vi "find_analog_data.vi"(10 "Needle":string, 11 "Haystack":T1[](array[typedef])) -> (0 "Index":i32, 1 "Found?":bool, 2 "Needle Out":T1)   [LabVIEW 2017]
uses:
  Box/Annular Flow/Jason/LabVIEW 2017/Input Channel Lists/analog_data.ctl
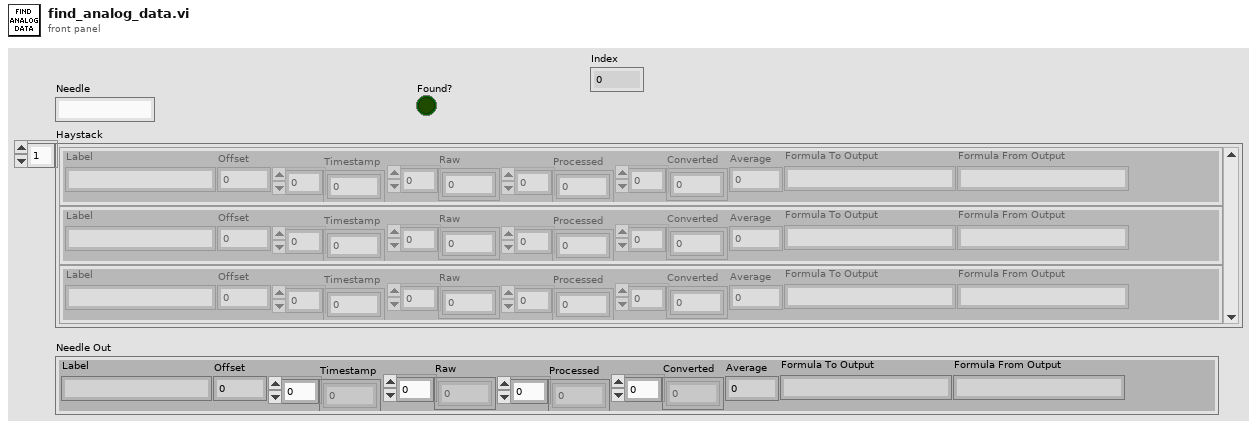
[diagram p1: front panel]
types:
  T1 = typedef "analog_data.ctl" = cluster{"Label":string, "Offset":dbl, "Timestamp":dbl[], "Raw":dbl[], "Processed":dbl[], "Converted":dbl[], "Average":dbl, "Formula To Output":string, "Formula From Output":string}
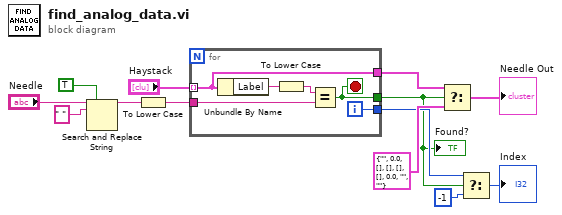
[diagram p0: block diagram]
diagram:
  n1 = Search and Replace String(replace all?=TRUE ("replace all? (F)"), input string="Needle", search string=" ") -> (result string=w9:string)  [unwired: 5 in, 3 out]
  n2 = To Lower Case(string=w9) -> (all lower case string=w8:string)
  n3 = for {
    tunnel: "Haystack" -> [w15] mode=indexing
    tunnel: w8 -> [w17]
    tunnel: [w16] -> w2
    tunnel: [w15] -> w7
    tunnel: [w14] -> w3
    i -> [w14]
    stop <- w16 stop-if-true
    n4 = Unbundle By Name(w15) -> ("Label"=w19:string)
    n5 = To Lower Case(string=w19) -> (all lower case string=w18:string)
    n6 = Equal?(x=w18, y=w17) -> (x = y?=w16:bool)
  }
  "Found?" <- w2
  n7 = Select(t=w7, s=w2, f=T1 {"Label"="", "Offset"=0.0, "Timestamp"=[], "Raw"=[], "Processed"=[], "Converted"=[], "Average"=0.0, "Formula To Output"="", "Formula From Output"=""}) -> (s? t:f=→"Needle Out":T1)
  n8 = Select(t=w3, s=w2, f=-1) -> (s? t:f=→"Index":i32)
